vi "CIMAQ_WindowArray.vi"(10 "Size":i32=5, 11 "Src":T1) -> (0 "error out":errorcluster, 2 "Image Pixels (U8)":u8[][](array[numeric]), 3 "Windows":u8[][][][](array[numeric]))   [LabVIEW 2017]
uses:
  <vilib>/vision/Image Controls.llb/IMAQ Image.ctl
  <vilib>/vision/EDVR.llb/IMAQ ImageToEDVR 2D U8.vi
  <vilib>/vision/NI_Vision_Development_Module.lvlib
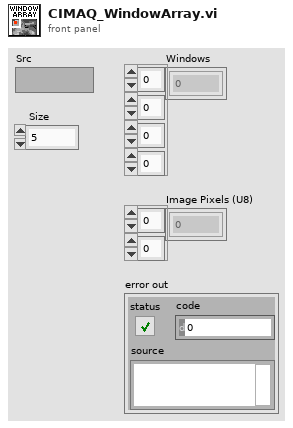
[diagram p1: front panel]
types:
  T1 = typedef "IMAQ Image.ctl" = refnum<image>
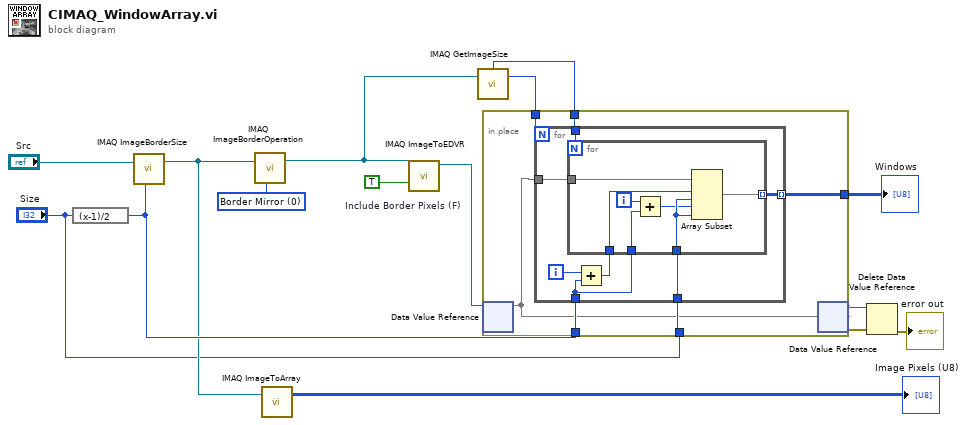
[diagram p0: block diagram]
diagram:
  w6 = u32 0 items=["Border Mirror", "Border Copy", "Border Clear"] ("Function")
  w1 = TRUE  # Include Border Pixels (F)
  n1 = expression code="(x-1)/2"("Size") -> (w13:i32)
  n2 = call "IMAQ ImageBorderSize"("Image"="Src", "Image border size in"=w13) -> ("Image Out"=w12:T1)  [unwired: 2 in, 2 out]
  n3 = call "IMAQ ImageBorderOperation"("Image"=w12, "Function"=w6) -> ("Image Out"=w5:T1)  [unwired: 3 in, 1 out]
  n4 = call "IMAQ ImageToArray"("Image"=w12) -> ("Image Pixels (U8)"=→"Image Pixels (U8)":u8[][])  [unwired: 3 in, 4 out]
  n5 = call-poly <vilib>:"IMAQ ImageToEDVR.vi"("Include Border Pixels (F)"=w1, "Image"=w5) -> ("EDVR 2D U8"=w2:refnum<data-value>)  [unwired: 7 in, 2 out]
  n6 = call "IMAQ GetImageSize"("Image"=w5) -> ("Y Resolution"=w3:i32, "X Resolution"=w4:i32)  [unwired: 3 in, 1 out]
  n7 = in-place {
    in-place-border: "Size" -> [w21]
    in-place-border: w13 -> [w20]
    in-place-border: w3 -> [w19]
    in-place-border: w4 -> [w18]
    in-place-border: [w17] -> w10
    n8 = in-place-dvr #1(w2) -> (w16:u8[][])  [unwired: 1 out]
    n9 = for {
      N: w19 -> [_]
      tunnel: w16 -> [w28]
      tunnel: w21 -> [w24]
      tunnel: w20 -> [w22]
      tunnel: w18 -> [w27]
      tunnel: [w25] -> w17 mode=indexing
      i -> [w23]
      n10 = Add(x=w23, y=w22) -> (x+y=w26:i32)
      n11 = for {
        N: w27 -> [_]
        tunnel: w28 -> [w35]
        tunnel: w24 -> [w34]
        tunnel: w26 -> [w33]
        tunnel: w22 -> [w30]
        tunnel: [w29] -> w25 mode=indexing
        i -> [w32]
        n12 = Add(x=w32, y=w30) -> (x+y=w31:i32)
        n13 = Array Subset "Array Subset"(array=w35, index (row)=w33, length (row)=w34, index (col)=w31, length (col)=w34) -> (w29:u8[][])
      }
    }
    n14 = in-place-dvr #1(w16) -> (w8:refnum<data-value>, w14:errorcluster)
  }
  "Windows" <- w10
  n15 = Delete Data Value Reference(data value reference=w8, error in=w14) -> (error out=→"error out":errorcluster)  [unwired: 1 out]
